vi "PIXY Publisher.vi"(6 "Brightness":u8(slide)=80 scale=0.0..255.0, 7 "Color Combo Object":T1(array[cluster]), 8 "Color":cluster{"Red":u8, "Green":u8, "Blue":u8} {"Blue" scale=0.0..255.0; "Green" scale=0.0..255.0; "Red" scale=0.0..255.0}, 9 "TimeStamp in":u32, 10 "Object":T2(array[cluster]), 11 "Operation":T3(ring)) -> (0 "Color Out":cluster{"Red":u8, "Green":u8, "Blue":u8} {"Blue" scale=0.0..255.0; "Green" scale=0.0..255.0; "Red" scale=0.0..255.0}, 1 "TimeStamp out":u32, 2 "Object Out":T2(array[cluster]), 4 "Brightness Out":u8(slide)=80 scale=0.0..255.0, 5 "Color Combo Object Out":T1(array[cluster]))   [LabVIEW 2016]
doc: "Use this to store and retrieve the properties of the PIXY camera. The communications loop will access the data that needs to be sent to the camera and will store the most recent objects here."
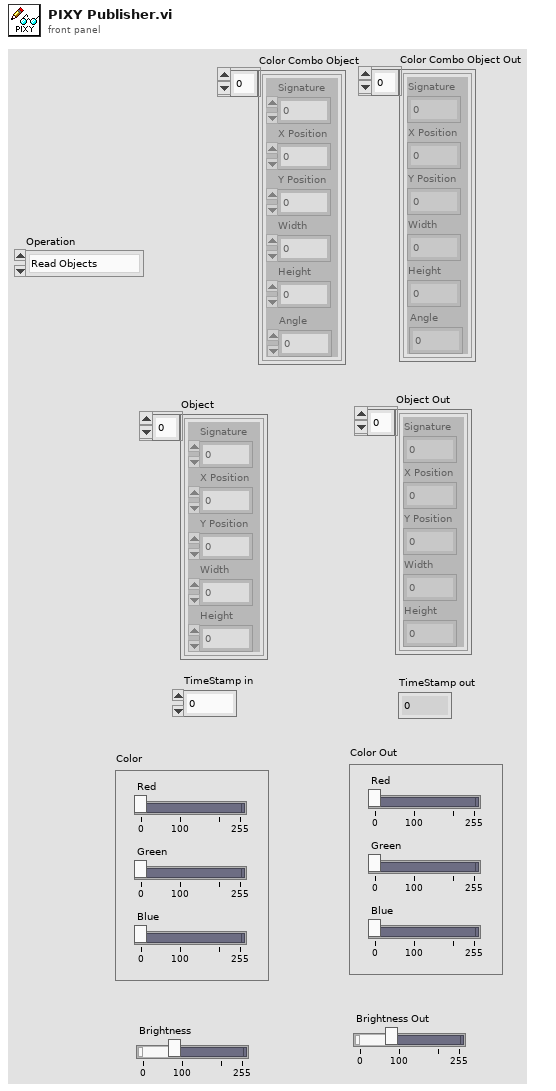
[diagram p1: front panel]
types:
  T1 = cluster{"Signature":u16, "X Position":u16, "Y Position":u16, "Width":u16, "Height":u16, "Angle":i16}[]
  T2 = cluster{"Signature":u16, "X Position":u16, "Y Position":u16, "Width":u16, "Height":u16}[]
  T3 = enum16{"Read Objects", "Write LED Color", "Write Brightness", "Write Objects", "Read Settings", "Clear"}
  T4 = cluster{"Object":cluster{"Signature":u16, "X Position":u16, "Y Position":u16, "Width":u16, "Height":u16}[], "TimeStamp in":u32, "Brightness":u8, "Color":cluster{"Red":u8, "Green":u8, "Blue":u8}, "CC Object":cluster{"Signature":u16, "X Position":u16, "Y Position":u16, "Width":u16, "Height":u16, "Height 2":i16}[]}
  T5 = cluster{"Signature":u16, "X Position":u16, "Y Position":u16, "Width":u16, "Height":u16, "Height 2":i16}[]
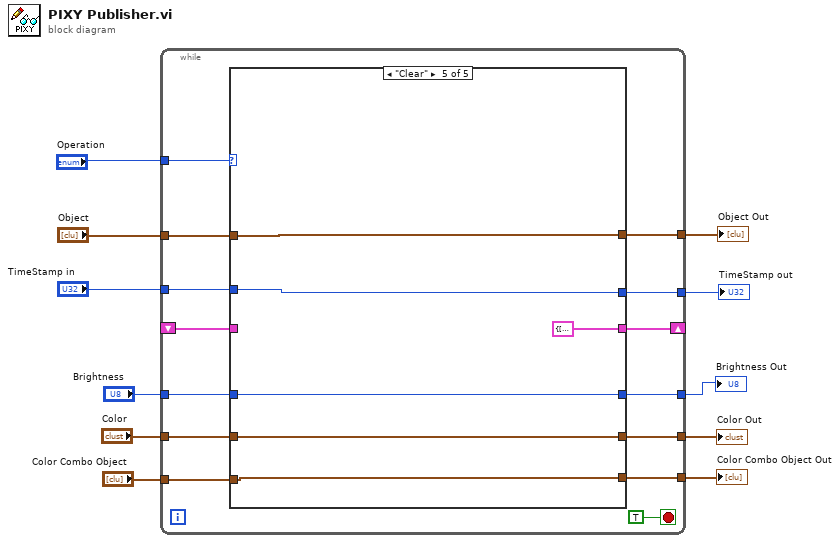
[diagram p0: block diagram]
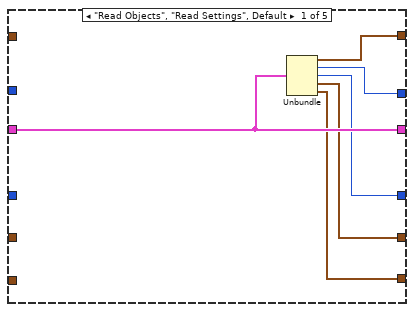
[diagram p2: hidden frame]
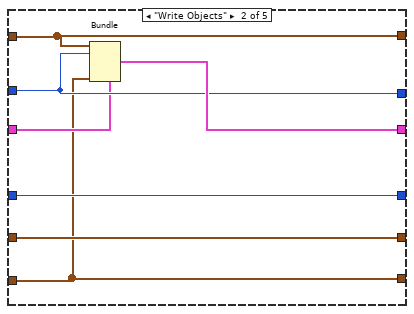
[diagram p3: hidden frame]
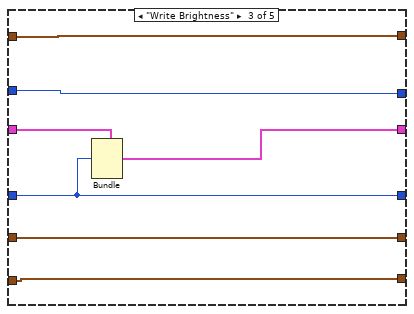
[diagram p4: hidden frame]
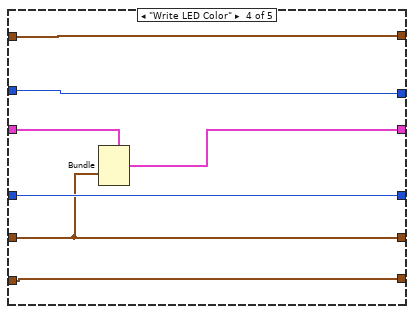
[diagram p5: hidden frame]
diagram:
  n1 = while {
    tunnel: "Operation" -> [w24]
    tunnel: "Object" -> [w23]
    tunnel: "TimeStamp in" -> [w22]
    shift-right: [w21] -> _
    shift-left: _ -> [w20]
    tunnel: [w19] -> w8
    tunnel: [w18] -> w7
    tunnel: "Brightness" -> [w17]
    tunnel: [w16] -> w5
    tunnel: "Color" -> [w15]
    tunnel: [w14] -> w3
    tunnel: [w13] -> w2
    tunnel: "Color Combo Object" -> [w12]
    stop <- TRUE stop-if-true
    n2 = case shown="\"Clear\"" w24 {
      tunnel: w23 -> [_ w37 w44 w51 w58]
      tunnel: w22 -> [_ w36 w43 w50 w57]
      tunnel: [w29 w38 w45 w52 T4 {"Object"=[], "TimeStamp in"=0, "Brightness"=0, "Color"={"Red"=0, "Green"=0, "Blue"=0}, "CC Object"=[]}] -> w21
      tunnel: w20 -> [w29 w35 w42 w49 _]
      tunnel: [w31 w37 w44 w51 w58] -> w19
      tunnel: [w30 w36 w43 w50 w57] -> w18
      tunnel: w17 -> [_ w34 w40 w48 w56]
      tunnel: [w27 w33 w41 w47 w55] -> w16
      tunnel: w15 -> [_ w33 w41 w47 w55]
      tunnel: [w28 w34 w40 w48 w56] -> w14
      tunnel: [w26 w32 w39 w46 w54] -> w13
      tunnel: w12 -> [_ w32 w39 w46 w54]
      frame "Read Objects", "Read Settings", Default {
        n3 = Unbundle(w29) -> ("Object"=w31:T2, "TimeStamp in"=w30:u32, "Brightness"=w28:u8, "Color"=w27:cluster{"Red":u8, "Green":u8, "Blue":u8}, "CC Object"=w26:T5)
      }
      frame "Write Objects" {
        n4 = Bundle(cluster=w35, "Object"=w37, "TimeStamp in"=w36, "CC Object"=w32) -> (w38:T4)  [unwired: 2 in]
      }
      frame "Write Brightness" {
        n5 = Bundle(cluster=w42, "Brightness"=w40) -> (w45:T4)  [unwired: 4 in]
      }
      frame "Write LED Color" {
        n6 = Bundle(cluster=w49, "Color"=w47) -> (w52:T4)  [unwired: 4 in]
      }
      frame "Clear" {
      }
    }
  }
  "Object Out" <- w8
  "TimeStamp out" <- w7
  "Color Out" <- w5
  "Brightness Out" <- w3
  "Color Combo Object Out" <- w2
